vi "iPScontrol_Ethernet.vi"() -> ()   [LabVIEW 2014]
panel:
  out "Set Field":string
  out "Switch Heater":string
  out "STATUS":string
  out "He level":string
  out "Reading of persistant field":string
  in  "error in (no error)":errorcluster
  out "error out":errorcluster
  out "Reading of magnetic field":string
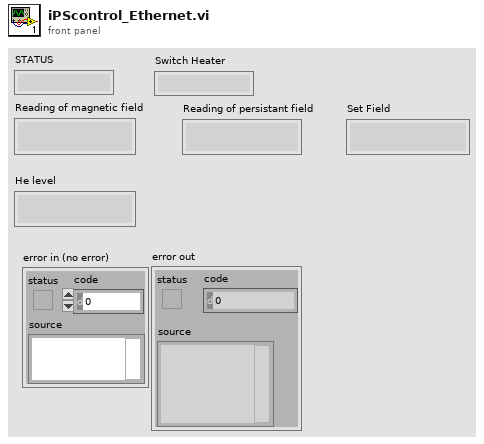
[diagram p1: front panel]
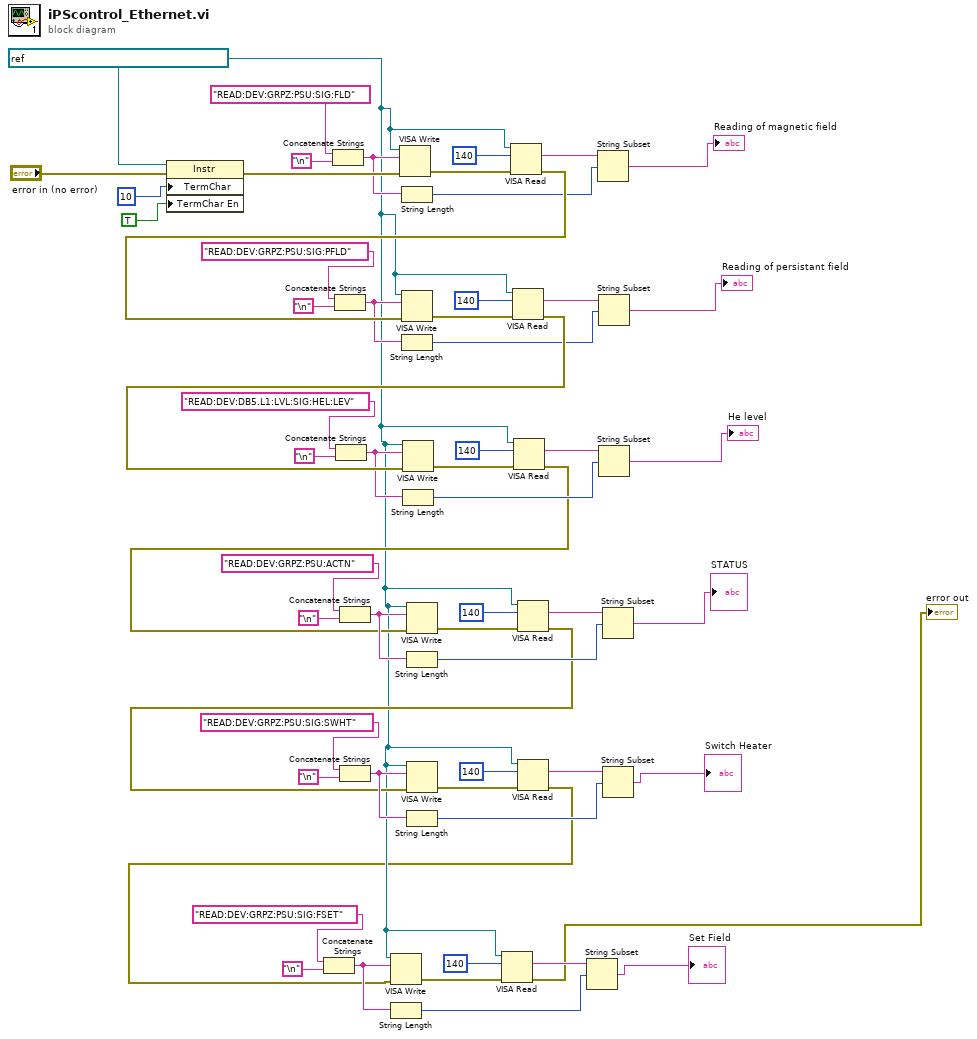
[diagram p0: block diagram]
diagram:
  w3 = refnum<visa-resource-name> "TCPIP0::192.168.128.3::7020::SOCKET" ("VISA resource name")
  n1 = property class="Instr"(reference=w3, error in="error in (no error)", "TermChar"=10, "TermChar En"=TRUE) -> (error out=w48:errorcluster)  [unwired: 1 out]
  n2 = Concatenate Strings("READ:DEV:GRPZ:PSU:SIG:FSET" ("string"), "\n") -> (w5:string)
  n3 = Concatenate Strings("READ:DEV:GRPZ:PSU:SIG:FLD" ("string"), "\n") -> (w41:string)
  n4 = Concatenate Strings("READ:DEV:GRPZ:PSU:SIG:PFLD" ("string"), "\n") -> (w34:string)
  n5 = Concatenate Strings("READ:DEV:DB5.L1:LVL:SIG:HEL:LEV" ("string"), "\n") -> (w30:string)
  n6 = Concatenate Strings("READ:DEV:GRPZ:PSU:ACTN" ("string"), "\n") -> (w23:string)
  n7 = Concatenate Strings("READ:DEV:GRPZ:PSU:SIG:SWHT" ("string"), "\n") -> (w15:string)
  n8 = String Length(string=w5) -> (length=w6:i32)
  n9 = VISA Write(VISA resource name=w3, write buffer=w41, error in (no error)=w48) -> (error out=w59:errorcluster)  [unwired: 2 out]
  n10 = String Length(string=w41) -> (length=w38:i32)
  n11 = String Length(string=w34) -> (length=w35:i32)
  n12 = String Length(string=w30) -> (length=w31:i32)
  n13 = String Length(string=w23) -> (length=w24:i32)
  n14 = String Length(string=w15) -> (length=w16:i32)
  n15 = VISA Read(VISA resource name=w3, byte count=140, error in (no error)=w59) -> (read buffer=w40:string, error out=w50:errorcluster)  [unwired: 2 out]
  n16 = VISA Write(VISA resource name=w3, write buffer=w34, error in (no error)=w50) -> (error out=w54:errorcluster)  [unwired: 2 out]
  n17 = VISA Read(VISA resource name=w3, byte count=140, error in (no error)=w54) -> (read buffer=w36:string, error out=w42:errorcluster)  [unwired: 2 out]
  n18 = VISA Write(VISA resource name=w3, write buffer=w30, error in (no error)=w42) -> (error out=w46:errorcluster)  [unwired: 2 out]
  n19 = VISA Read(VISA resource name=w3, byte count=140, error in (no error)=w46) -> (read buffer=w32:string, error out=w22:errorcluster)  [unwired: 2 out]
  n20 = VISA Write(VISA resource name=w3, write buffer=w23, error in (no error)=w22) -> (error out=w29:errorcluster)  [unwired: 2 out]
  n21 = VISA Read(VISA resource name=w3, byte count=140, error in (no error)=w29) -> (read buffer=w25:string, error out=w14:errorcluster)  [unwired: 2 out]
  n22 = VISA Write(VISA resource name=w3, write buffer=w15, error in (no error)=w14) -> (error out=w21:errorcluster)  [unwired: 2 out]
  n23 = VISA Read(VISA resource name=w3, byte count=140, error in (no error)=w21) -> (read buffer=w17:string, error out=w2:errorcluster)  [unwired: 2 out]
  n24 = VISA Write(VISA resource name=w3, write buffer=w5, error in (no error)=w2) -> (error out=w11:errorcluster)  [unwired: 2 out]
  n25 = VISA Read(VISA resource name=w3, byte count=140, error in (no error)=w11) -> (read buffer=w7:string, error out=→"error out":errorcluster)  [unwired: 2 out]
  n26 = String Subset(string=w7, offset (0)=w6) -> (substring=→"Set Field":string)  [unwired: 1 in]
  n27 = String Subset(string=w40, offset (0)=w38) -> (substring=→"Reading of magnetic field":string)  [unwired: 1 in]
  n28 = String Subset(string=w36, offset (0)=w35) -> (substring=→"Reading of persistant field":string)  [unwired: 1 in]
  n29 = String Subset(string=w32, offset (0)=w31) -> (substring=→"He level":string)  [unwired: 1 in]
  n30 = String Subset(string=w25, offset (0)=w24) -> (substring=→"STATUS":string)  [unwired: 1 in]
  n31 = String Subset(string=w17, offset (0)=w16) -> (substring=→"Switch Heater":string)  [unwired: 1 in]
